vi "FTW-Ether-Address-Validate.vi"(5 "Address":T1, 11 "error in":errorcluster) -> (6 "Sanitized Address":T1, 8 "Message Transport Scheme":T2, 15 "error out":errorcluster)   [LabVIEW 2012, in "FTW-Actor.lvlib" / "FTW-Ether.lvclass"]
uses:
  FTW-Ether.lvclass
  Utility/FTW-Actor-Address.ctl
  FTW-Ether-MessageTransportScheme.ctl
  Core/src/Error/FTW-ERR-ThrowError.vi
  FTW-Actor.lvlib
panel:
  # "Inputs"
  # "Outputs"
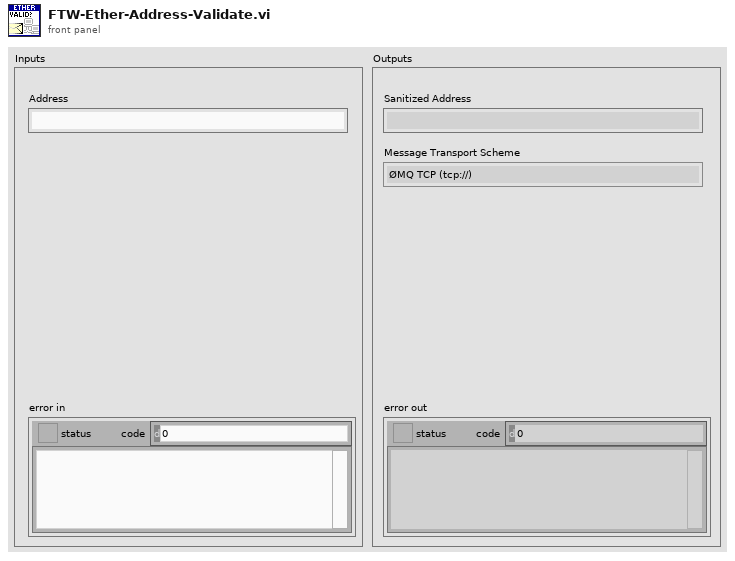
[diagram p1: front panel]
types:
  T1 = typedef "FTW-Actor.lvlib/FTW-Actor-Address.ctl" = string
  T2 = typedef "FTW-Actor.lvlib/FTW-Ether.lvclass/FTW-Ether-MessageTransportScheme.ctl" = enum16{"ØMQ TCP (tcp://)", "ØMQ In-Process (inproc://)", "LabVIEW Queues (lvq://)", "LabVIEW Network Streams (lvns://)"}
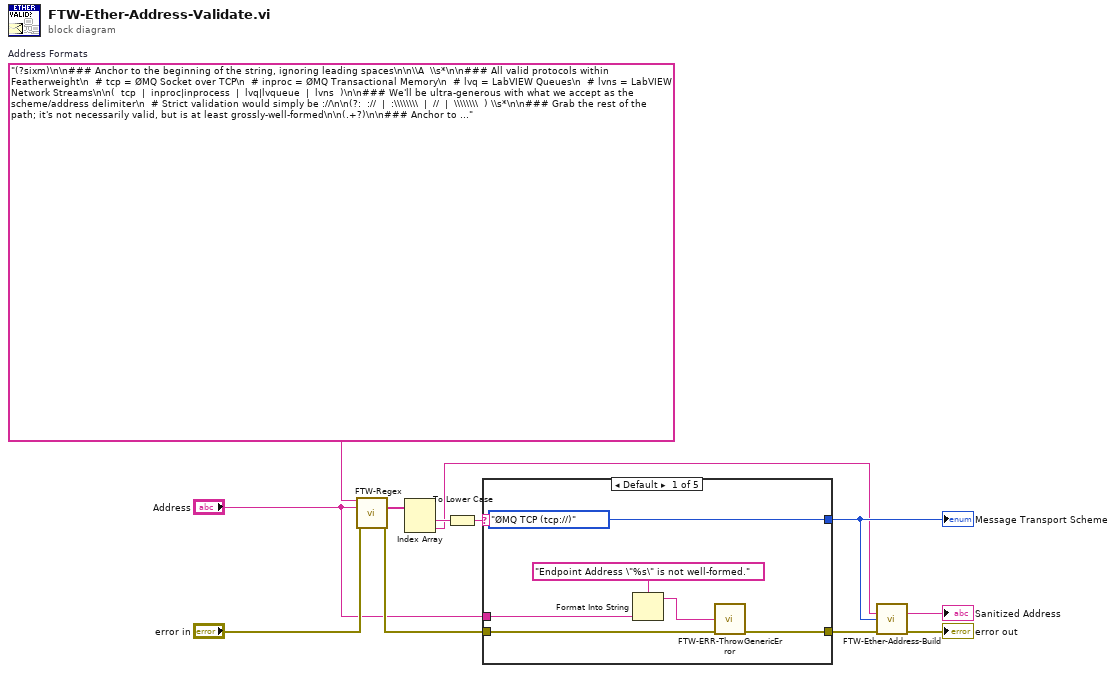
[diagram p0: block diagram]
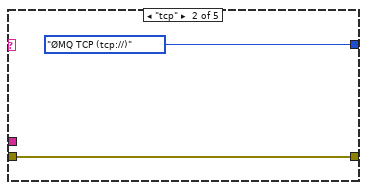
[diagram p2: hidden frame]
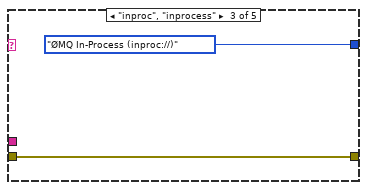
[diagram p3: hidden frame]
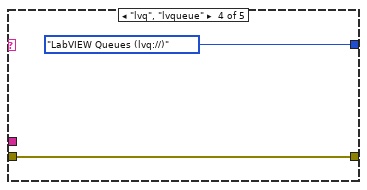
[diagram p4: hidden frame]
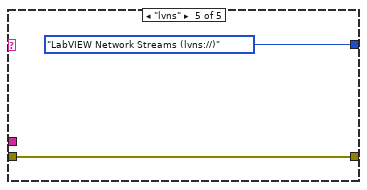
[diagram p5: hidden frame]
diagram:
  w12 = "(?sixm)\n\n### Anchor to the beginning of the string, ignoring leading spaces\n\n\\A  \\s*\n\n### All valid protocols within Featherweight\n  # tcp = ØMQ Socket over TCP\n  # inproc = ØMQ Transactional Memory\n  # lvq = LabVIEW Queues\n  # lvns = LabVIEW Network Streams\n\n(  tcp  |  inproc|inprocess  |  lvq|lvqueue  |  lvns  )\n\n### We'll be ultra-generous with what we accept as the scheme/address delimiter\n  # Strict validation would simply be ://\n\n(?:  ://  |  :\\\\\\\\  |  //  |  \\\\\\\\  ) \\s*\n\n### Grab the rest of the path; it's not necessarily valid, but is at least grossly-well-formed\n\n(.+?)\n\n### Anchor to the end of the string, ignoring trailing spaces\n\\s*\\z"  # Address Formats
  n1 = call "FTW-Regex.vi"("Regular Expression"=w12, "Input String"="Address", "error in"="error in") -> ("Submatches"=w11:string[], "error out"=w7:errorcluster)  [unwired: 8 in, 3 out]
  n2 = Index Array(array=w11) -> (element #1=w9:string, element #2=w1:string)  [unwired: 2 in]
  n3 = To Lower Case(string=w9) -> (all lower case string=w8:string)
  n4 = case shown="Default" w8 {
    tunnel: [FTW-Ether-MessageTransportScheme."ØMQ TCP (tcp://)" ("Message Transport Scheme") FTW-Ether-MessageTransportScheme."ØMQ TCP (tcp://)" ("Message Transport Scheme") FTW-Ether-MessageTransportScheme."ØMQ In-Process (inproc://)" ("Message Transport Scheme") FTW-Ether-MessageTransportScheme."LabVIEW Queues (lvq://)" ("Message Transport Scheme") FTW-Ether-MessageTransportScheme."LabVIEW Network Streams (lvns://)" ("Message Transport Scheme")] -> w2
    tunnel: w7 -> [w15 w19 w21 w23 w25]
    tunnel: "Address" -> [w14 _ _ _ _]
    tunnel: [w13 w19 w21 w23 w25] -> w3
    frame Default {
      n5 = Format Into String(format string="Endpoint Address \"%s\" is not well-formed." ("Error Message"), w14) -> (resulting string=w17:string)  [unwired: 2 in, 1 out]
      n6 = call "FTW-ERR-ThrowGenericError.vi"("Error Message"=w17, "error in"=w15) -> ("error out"=w13:errorcluster)  [unwired: 13 in]
    }
    frame "tcp" {
    }
    frame "inproc", "inprocess" {
    }
    frame "lvq", "lvqueue" {
    }
    frame "lvns" {
    }
  }
  "Message Transport Scheme" <- w2
  n7 = call "FTW-Ether-Address-Build.vi"("Path"=w1, "Message Transport Scheme"=w2, "error in"=w3) -> ("Endpoint Address"=→"Sanitized Address":T1, "error out"=→"error out":errorcluster)  [unwired: 11 in]
